vi "PopupDuplicationDictionnaire.vi"(8 "error in (no error)":errorcluster) -> (0 "error out":errorcluster, 2 "Nouveau dictionnaire Out":string, 3 "Edition annulée ?":bool)   [LabVIEW 2010]
uses:
  030 - EVENTS/EnumFgvEventCommand.ctl
  090 - ERRORS/Ctrls/enumLogAndView.ctl
  080 - TOOLS/Traduction/Dictionnary/EnumCommandDictionnaire.ctl
  030 - EVENTS/02 - ToScreens/ToScreensCommand.ctl
panel:
  out "Logo 600 X 200":picture
  in  "Nouveau dictionnaire":string
  out "Dictionnaire courant":string
  in  "Bouton Enregistrer":bool
  in  "BoutonQuitter":bool
  # "Duplication dictionnaire"
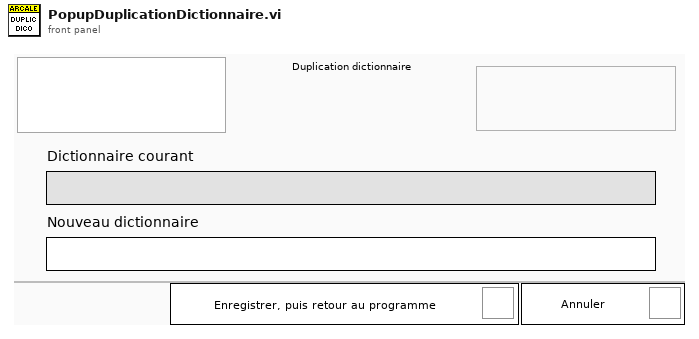
[diagram p1: front panel]
types:
  T1 = typedef "EnumFgvEventCommand.ctl" = enum16{"Setup", "Cleanup", "Get"}
  T2 = typedef "EnumCommandDictionnaire.ctl" = enum16{"Load", "Translate", "Save", "GetDico", "Set : A traduire = Vrai", "Set : A Traduire = Faux", "SetDico"}
  T3 = enum8{"Enabled", "Disabled", "Disabled and Grayed Out"}
  T4 = typedef "ApplicationInfos.ctl" = cluster{"ApplicationName":string, "ApplicationVersion":string, "Logo 600X200 path":path, "Logo 400X400 path":path, "Client":string}
  T5 = typedef "Dictionnaire.ctl" = cluster{"FichierDictionnaire":path, "TabCleValeur":T6[], "DictionnaireModifié?":bool, "Traduction à réaliser ?":bool, "Interdire l'ajout de nouvelles clés ?":bool}
  T6 = typedef "CleValeur.ctl" = cluster{"Clé":string, "Valeur":string}
  T7 = typedef "enumLogAndView.ctl" = enum16{"Log only", "Log and view"}
  T8 = typedef "ToScreensCommand.ctl" = enum16{"Stop screen", "Stop all screens"}
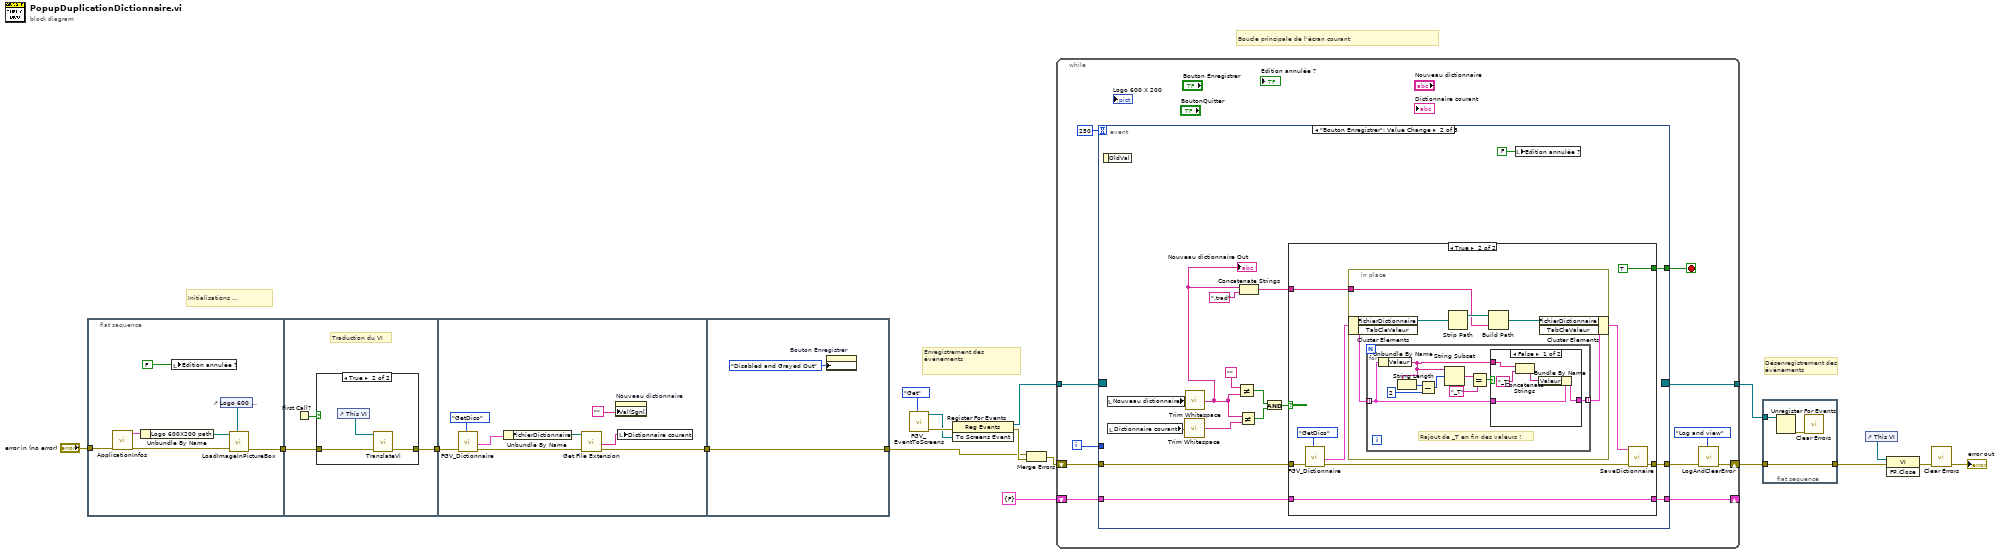
[diagram p0: block diagram]
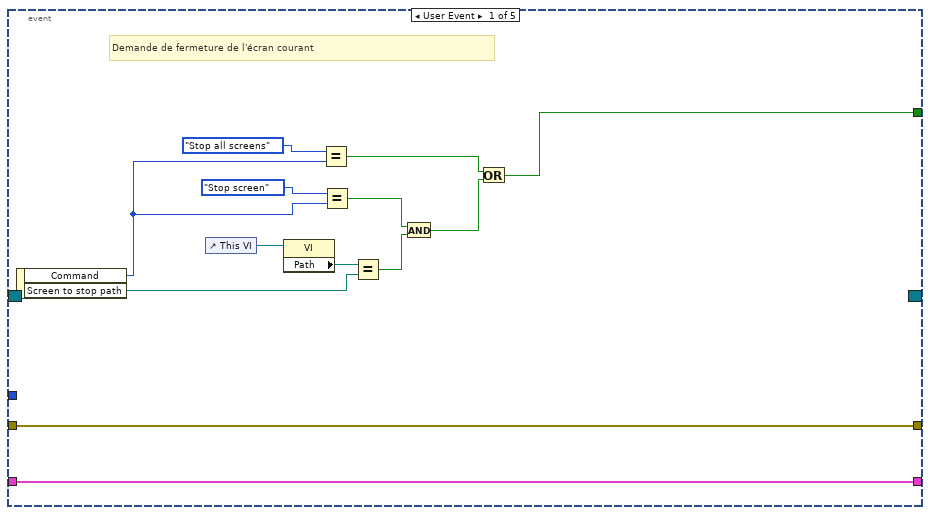
[diagram p3: hidden frame]
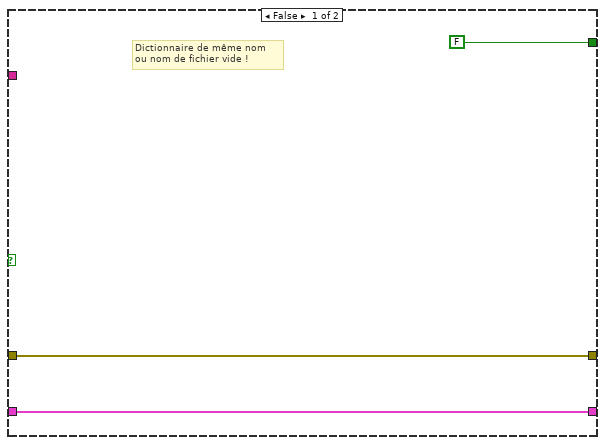
[diagram p4: hidden frame]
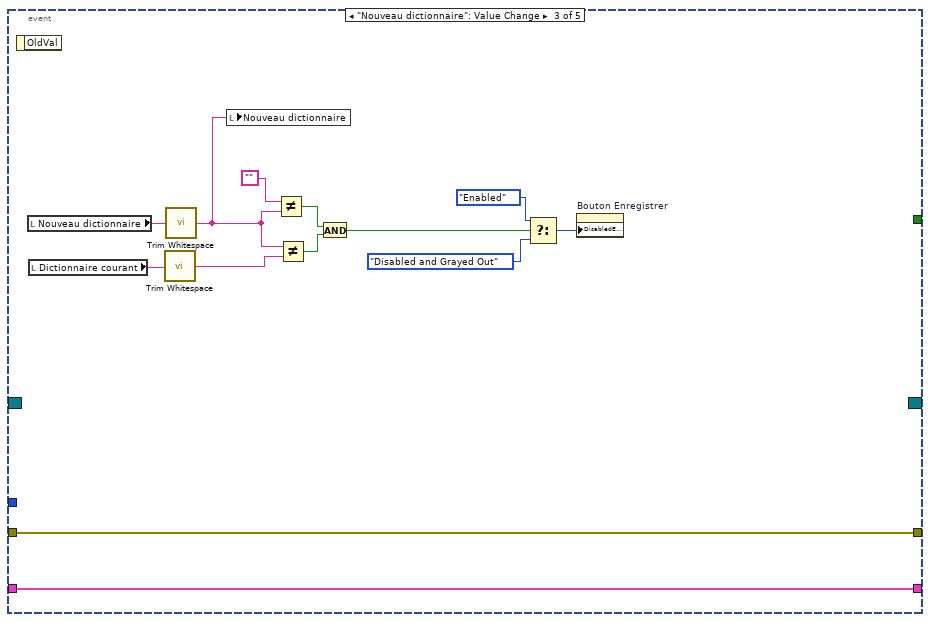
[diagram p6: hidden frame]
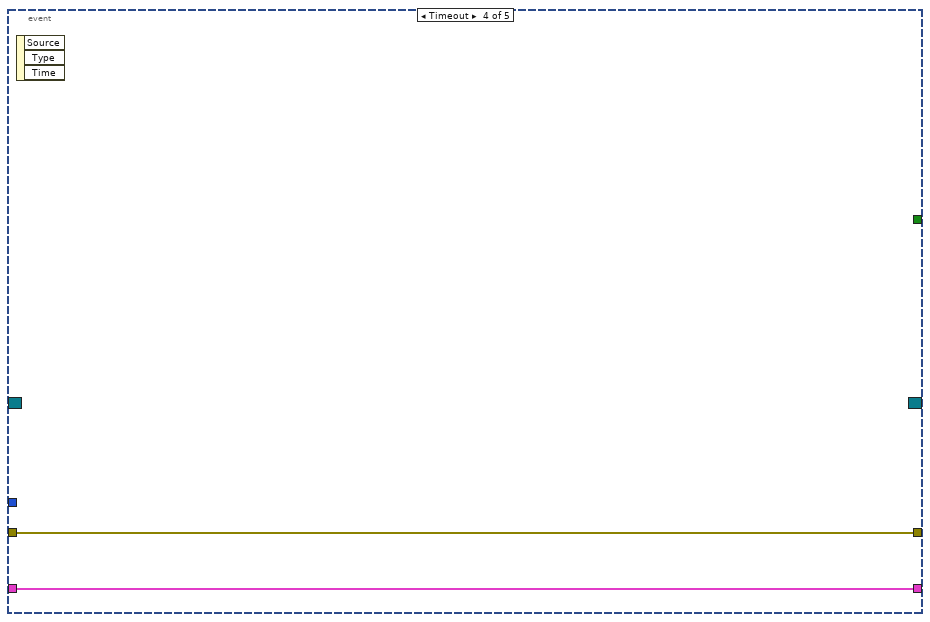
[diagram p7: hidden frame]
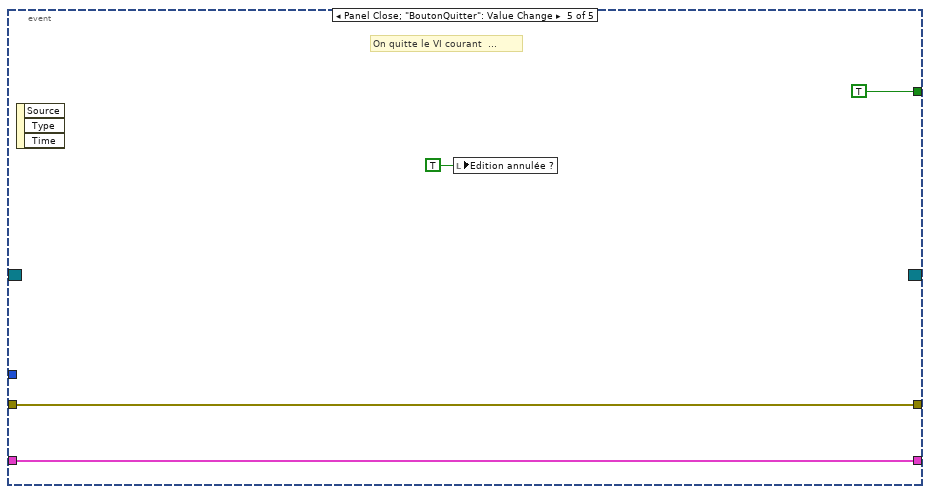
[diagram p8: hidden frame]
diagram:
  # "Initialisations ..."
  # "Boucle principale de l'écran courant"
  # "Désenregistrement des \névénements"
  # "Enregistrement des \névénements"
  n1 = flat-sequence {
    tunnel: "error in (no error)" -> [w21]
    tunnel: [w20] -> w5
    tunnel: w5 -> [w27]
    tunnel: [w28] -> w4
    tunnel: w4 -> [w40]
    tunnel: [w35] -> w3
    tunnel: w3 -> [w41]
    tunnel: [w41] -> w2
    frame #0 {
      n2 = call "ApplicationInfos.vi"("error in (no error)"=w21) -> ("error out"=w25:errorcluster, "ApplicationInfo"=w23:T4)  [unwired: 9 in]
      n3 = Unbundle By Name(w23) -> ("Logo 600X200 path"=w22:path)
      n4 = local write "Edition annulée ?"(FALSE ("Suppression confirmée ?")) -> ()
      n5 = control-ref of="Logo 600 X 200"() -> (w24:refnum<vi>)
      n6 = call "LoadImageInPictureBox.vi"("Pict Refnum In"=w24, "error in (no error)"=w25, "Image file path"=w22) -> ("error out"=w20:errorcluster)  [unwired: 8 in]
    }
    frame #1 {
      # "Traduction du VI"
      n7 = First Call?() -> (First Call?: T/F=w26:bool)
      n8 = case shown="True" w26 {
        tunnel: [w29 w32] -> w28
        tunnel: w27 -> [w29 w30]
        frame False {
        }
        frame True {
          n9 = control-ref of="This VI"() -> (w31:refnum<vi>)
          n10 = call "TranslateVi.vi"("error in (no error)"=w30, "VI ref"=w31) -> ("error out"=w32:errorcluster)  [unwired: 9 in]
        }
      }
    }
    frame #2 {
      n11 = call "FGV_Dictionnaire.vi"("Command"=EnumCommandDictionnaire."GetDico", "error in (no error)"=w40) -> ("error out"=w36:errorcluster, "Dictionnaire Out"=w38:T5)  [unwired: 7 in, 1 out]
      n12 = Unbundle By Name(w38) -> ("FichierDictionnaire"=w37:path)
      n13 = call <vilib>:"Get File Extension.vi"("error in (no error)"=w36, "file"=w37) -> ("error out"=w35:errorcluster, "filename without extension"=w34:string)  [unwired: 6 in, 2 out]
      n14 = property on="Nouveau dictionnaire" class="Str"("Val(Sgnl)"="") -> ()  [unwired: 2 in, 2 out]
      n15 = local write "Dictionnaire courant"(w34) -> ()
    }
    frame #3 {
      n16 = property on="Bouton Enregistrer" class="Bool"("DisabledEnum"=T3."Disabled and Grayed Out" ("Disabled")) -> ()  [unwired: 2 in, 2 out]
    }
  }
  n17 = call "FGV_EventToScreens.vi"("Command"=EnumFgvEventCommand."Get") -> ("error out"=w15:errorcluster, "To Screens Event"=w13:refnum<user-event>)  [unwired: 9 in]
  n18 = register-events(error in=w15, w13) -> (reference out=w18:refnum<event-registration>, error out=w11:errorcluster)  [unwired: 1 in]
  n19 = Merge Errors(w2, w11) -> (w12:errorcluster)
  n20 = while {
    tunnel: w18 -> [w53]
    shift-right: [w45] -> w10
    shift-left: w12 -> [w52]
    tunnel: [w51] -> w9
    shift-right: [w49] -> _
    shift-left: cluster{"Boolean":bool} {"Boolean"=FALSE} ("appConfig") -> [w50]
    i -> [w47]
    stop <- w48 stop-if-true
    n21 = event shown="[1] \"Bouton Enregistrer\": Value Change" {
      selector: w53 -> [_ _ _ _ _]
      dyn-events: [_ _ _ _ _] -> w51
      timeout: 250 -> [_ _ _ _ _]
      tunnel: [w55 w71 _ _ TRUE ("stopCurrentScreen")] -> w48
      tunnel: w52 -> [w54 w75 w117 w130 w132]
      tunnel: [w54 w73 w117 w130 w132] -> w46
      tunnel: w50 -> [w66 w74 w116 w129 w133]
      tunnel: [w66 w72 w116 w129 w133] -> w49
      tunnel: w47 -> [_ _ _ _ _]
      event User Event {
        # "Demande de fermeture de l'écran courant"
        n22 = event-data() -> ("Command"=w63:T8, "Screen to stop path"=w60:path)  [unwired: 1 out]
        n23 = control-ref of="This VI"() -> (w62:refnum<vi>)
        n24 = property class="VI"(reference=w62) -> ("Path"=w61:path)  [unwired: 1 in, 2 out]
        n25 = Equal?(x=ToScreensCommand."Stop all screens", y=w63) -> (x = y?=w57:bool)
        n26 = Equal?(x=ToScreensCommand."Stop screen", y=w63) -> (x = y?=w59:bool)
        n27 = Equal?(x=w61, y=w60) -> (x = y?=w58:bool)
        n28 = And(x=w59, y=w58) -> (x .and. y?=w56:bool)
        n29 = Or(x=w57, y=w56) -> (x .or. y?=w55:bool)
      }
      event "Bouton Enregistrer": Value Change {
        n30 = event-data() -> ()  [unwired: 2 out]
        n31 = local read "Nouveau dictionnaire"() -> (w82:string)
        n32 = local read "Dictionnaire courant"() -> (w81:string)
        n33 = call <vilib>:"Trim Whitespace.vi"("string"=w81) -> ("trimmed string"=w80:string)  [unwired: 1 in]
        n34 = call <vilib>:"Trim Whitespace.vi"("string"=w82) -> ("trimmed string"=w68:string)  [unwired: 1 in]
        "Nouveau dictionnaire Out" <- w68
        n35 = Not Equal?(x="", y=w68) -> (x != y?=w77:bool)
        n36 = Not Equal?(x=w68, y=w80) -> (x != y?=w78:bool)
        n37 = Concatenate Strings(w68, ".trad" ("string")) -> (w69:string)
        n38 = And(x=w77, y=w78) -> (x .and. y?=w76:bool)
        n39 = case shown="True" w76 {
          tunnel: w75 -> [w85 w92]
          tunnel: w74 -> [w84 w94]
          tunnel: [w85 w90] -> w73
          tunnel: [w84 w94] -> w72
          tunnel: [FALSE ("stopCurrentScreen") TRUE ("stopCurrentScreen")] -> w71
          tunnel: w69 -> [_ w86]
          frame False {
            # "Dictionnaire de même nom\nou nom de fichier vide !"
          }
          frame True {
            n40 = call "FGV_Dictionnaire.vi"("Command"=EnumCommandDictionnaire."GetDico", "error in (no error)"=w92) -> ("error out"=w91:errorcluster, "Dictionnaire Out"=w88:T5)  [unwired: 7 in, 1 out]
            n41 = in-place {
              in-place-border: w86 -> [w98]
              n42 = in-place-cluster #1(w88) -> ("FichierDictionnaire"=w100:path, "TabCleValeur"=w96:T6[])
              n43 = for {
                tunnel: w96 -> [w108] mode=indexing
                tunnel: [w109] -> w95 mode=indexing
                # "Rajout de _T en fin des valeurs !"
                n44 = Unbundle By Name(w108) -> ("Valeur"=w101:string)
                n45 = String Length(string=w101) -> (length=w107:i32)
                n46 = Subtract(x=w107, y=2) -> (x-y=w105:i32)
                n47 = String Subset(string=w101, offset (0)=w105) -> (substring=w104:string)  [unwired: 1 in]
                n48 = Equal?(x=w104, y="_T") -> (x = y?=w102:bool)
                n49 = case shown="False" w102 {
                  tunnel: [w114 w115] -> w109
                  tunnel: w108 -> [w113 w115]
                  tunnel: w101 -> [w111 _]
                  frame False {
                    n50 = Concatenate Strings(w111, "_T") -> (w110:string)
                    n51 = Bundle By Name(cluster=w113, "Valeur"=w110) -> (w114:T6)
                  }
                  frame True {
                  }
                }
              }
              n52 = Strip Path(path=w100) -> (stripped path=w99:path)  [unwired: 1 out]
              n53 = Build Path(base path=w99, name or relative path=w98) -> (appended path=w97:path)
              n54 = in-place-cluster #1("FichierDictionnaire"=w97, "TabCleValeur"=w95) -> (w87:T5)
            }
            n55 = call "SaveDictionnaire.vi"("error in (no error)"=w91, "Dictionnaire"=w87) -> ("error out"=w90:errorcluster)  [unwired: 9 in]
          }
        }
        n56 = local write "Edition annulée ?"(FALSE ("Edition annulée ?")) -> ()
      }
      event "Nouveau dictionnaire": Value Change {
        n57 = event-data() -> ()  [unwired: 2 out]
        n58 = local read "Nouveau dictionnaire"() -> (w128:string)
        n59 = local read "Dictionnaire courant"() -> (w127:string)
        n60 = call <vilib>:"Trim Whitespace.vi"("string"=w127) -> ("trimmed string"=w126:string)  [unwired: 1 in]
        n61 = call <vilib>:"Trim Whitespace.vi"("string"=w128) -> ("trimmed string"=w118:string)  [unwired: 1 in]
        n62 = local write "Nouveau dictionnaire"(w118) -> ()
        n63 = Not Equal?(x="", y=w118) -> (x != y?=w123:bool)
        n64 = Not Equal?(x=w118, y=w126) -> (x != y?=w124:bool)
        n65 = And(x=w123, y=w124) -> (x .and. y?=w121:bool)
        n66 = Select(t=T3."Enabled" ("Disabled"), s=w121, f=T3."Disabled and Grayed Out" ("Disabled")) -> (s? t:f=w122:T3)
        n67 = property on="Bouton Enregistrer" class="Bool"("DisabledEnum"=w122) -> ()  [unwired: 2 in, 2 out]
      }
      event Timeout {
        n68 = event-data() -> ()  [unwired: 4 out]
      }
      event Panel Close; "BoutonQuitter": Value Change {
        # "On quitte le VI courant  ..."
        n69 = event-data() -> ()  [unwired: 4 out]
        n70 = local write "Edition annulée ?"(TRUE ("Edition annulée ?")) -> ()
      }
    }
    n71 = call "LogAndClearError.vi"("Log and view ?"=enumLogAndView."Log and view", "error in (no error)"=w46) -> ("error out"=w45:errorcluster)  [unwired: 9 in]
  }
  n72 = flat-sequence {
    tunnel: w9 -> [w137]
    tunnel: w10 -> [w135]
    tunnel: [w135] -> w1
    frame #0 {
      n73 = Unregister For Events(event registration refnum=w137) -> (error out=w136:errorcluster)  [unwired: 1 in]
      n74 = call <vilib>:"Clear Errors.vi"("error in (no error)"=w136) -> ()  [unwired: 7 out]
    }
  }
  n75 = control-ref of="This VI"() -> (w17:refnum<vi>)
  n76 = invoke class="VI" method="FP.Close"(reference=w17, error in=w1) -> (error out=w16:errorcluster)  [unwired: 1 in, 2 out]
  n77 = call <vilib>:"Clear Errors.vi"("error in (no error)"=w16) -> ("error out"=→"error out":errorcluster)  [unwired: 6 out]
